vi "Bar Page.vi"() -> ()   [LabVIEW 2017, in "3D Bar.lvclass"]
uses:
  <vilib>/Math Plots/3D Math Plots/3D Bar/3D Bar/3D Bar.lvclass
  <vilib>/Math Plots/3D Math Plots/3D Bar/3D Bar/Typedef/3D Bar Property Array.ctl
  <vilib>/Math Plots/3D Math Plots/3D Bar/3D Bar/Typedef/3D Bar Property.ctl
  <vilib>/Math Plots/3D Math Plots/3D Plot/3D Plot/Typedef/Line Type.ctl
  <vilib>/Math Plots/3D Math Plots/3D Plot/3D Plot/Typedef/Dialog State.ctl
  <vilib>/Math Plots/3D Math Plots/3D Plot/3D Plot/Typedef/Temp Scene State.ctl
  <vilib>/Math Plots/3D Math Plots/3D Plot/3D Plot/Typedef/Temp Scene Property Action.ctl
  <vilib>/Math Plots/3D Math Plots/3D Plot/3D Plot/3D Plot.lvclass
panel:
  in  "Bar Mode":u16(ring) caption="Bar mode" items=["Detach", "Group", "Stack"]
  in  "Line Style":u16(ring) caption="Line style"
  in  "Antialiasing":bool
  in  "Line Width":sgl=0.001 caption="Line width" min=0.001 step=1
  in  "Line Color":u32(colorbox) caption="Line color"
  in  "Color and Name":cluster{"Label Color":u32, "String":string}[](array[cluster]) caption="Color and name"
  in  "Bar Size":sgl=1.0 caption="Bar size" min=0.001 max=1 step=0.1
  out "Bar Property Out":T1
  in  "Bar Property In":T1
  in  "YZ Plane Projection":bool caption="YZ plane projection"
  in  "XZ Plane Projection":bool caption="XZ plane projection"
  in  "XY Plane Projection":bool caption="XY plane projection"
  in  "Coordinate System":u16(ring) caption="Coordinate system" items=["Cartesian", "Cylindrical", "Spherical"]
  in  "Plot Opacity":sgl(slide) caption="Plot opacity(%)" min=0 max=100 scale=0.0..100.0
  in  "Plot List":i32(listbox)
  in  "Move Down":bool
  in  "Move Up":bool
  in  "Delete":bool
  in  "New":bool
  in  "Event Registration":refnum<event-registration>
  # "Bar"
  # "General"
  # "Projection"
  # "Bar"
  # "Outline"
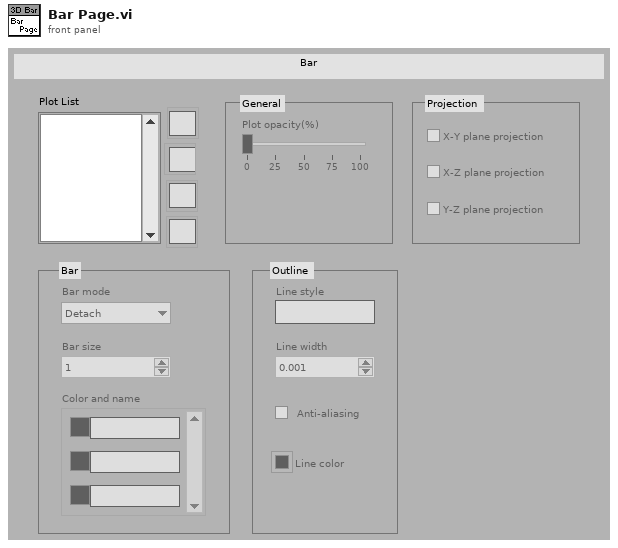
[diagram p1: front panel]
types:
  T1 = typedef "3D Bar.lvclass/3D Bar Property Array.ctl" = T2[]
  T2 = typedef "3D Bar.lvclass/3D Bar Property.ctl" = cluster{"General Property":cluster{"Plot Name":string, "Coordinate System":enum16{"Cartesian", "Cylindrical", "Spherical"}, "Opacity":sgl}, "Projection Property":cluster{"Draw XY":bool, "Draw YZ":bool, "Draw XZ":bool}, "Plot Property":cluster{"Line Style":T3, "Line Width":sgl, "Line Color":u32, "Antialiasing":bool}, "Bar Property":cluster{"Bar Mode":enum16{"Detach", "Group", "Stack"}, "Bar Width":sgl, "Color Pair Array":cluster{"Color":u32, "String":string}[]}}
  T3 = typedef "3D Plot.lvclass/Line Type.ctl" = enum16{"None", "Solid", "Dash", "Dot", "Dash Dot"}
  T4 = typedef "3D Plot.lvclass/Dialog State.ctl" = enum16{"Initialize", "Read Porperty", "Write Property", "Idle", "Exit"}
  T5 = typedef "3D Plot.lvclass/Temp Scene State.ctl" = enum16{"Create", "Update Scene", "Get Plot Representation", "Destory"}
  T6 = typedef "3D Plot.lvclass/Temp Scene Property Action.ctl" = enum16{"Graph Property", "Light Property", "Axis Property", "Value Pair Property", "Format Property", "Cursor Property", "Plot Specific Property"}
  T7 = typedef "3D Plot.lvclass/Multiplot Representation.ctl" = cluster{"Plot Represention Array":T8[], "Max Range":T9}
  T8 = typedef "3D Plot.lvclass/Plot Representation.ctl" = cluster{"Plot ID":i32, "Plot Range":T9, "Mesh Data":T10, "Dimension":cluster{"X Dimension":i32, "Y Dimension":i32}, "Ramp Range":T9}
  T9 = typedef "3D Plot.lvclass/Range Clusters.ctl" = cluster{"X Range":cluster{"Max X":sgl, "Min X":sgl}, "Y Range":cluster{"Max Y":sgl, "Min Y":sgl}, "Z Range":cluster{"Max Z":sgl, "Min Z":sgl}}
  T10 = typedef "3D Plot.lvclass/Mesh Data.ctl" = cluster{"Index Array":u32[], "Vertex Array":cluster{"X":sgl, "Y":sgl, "Z":sgl}[], "Normal Array":cluster{"X":sgl, "Y":sgl, "Z":sgl}[], "Color Index Array":i32[]}
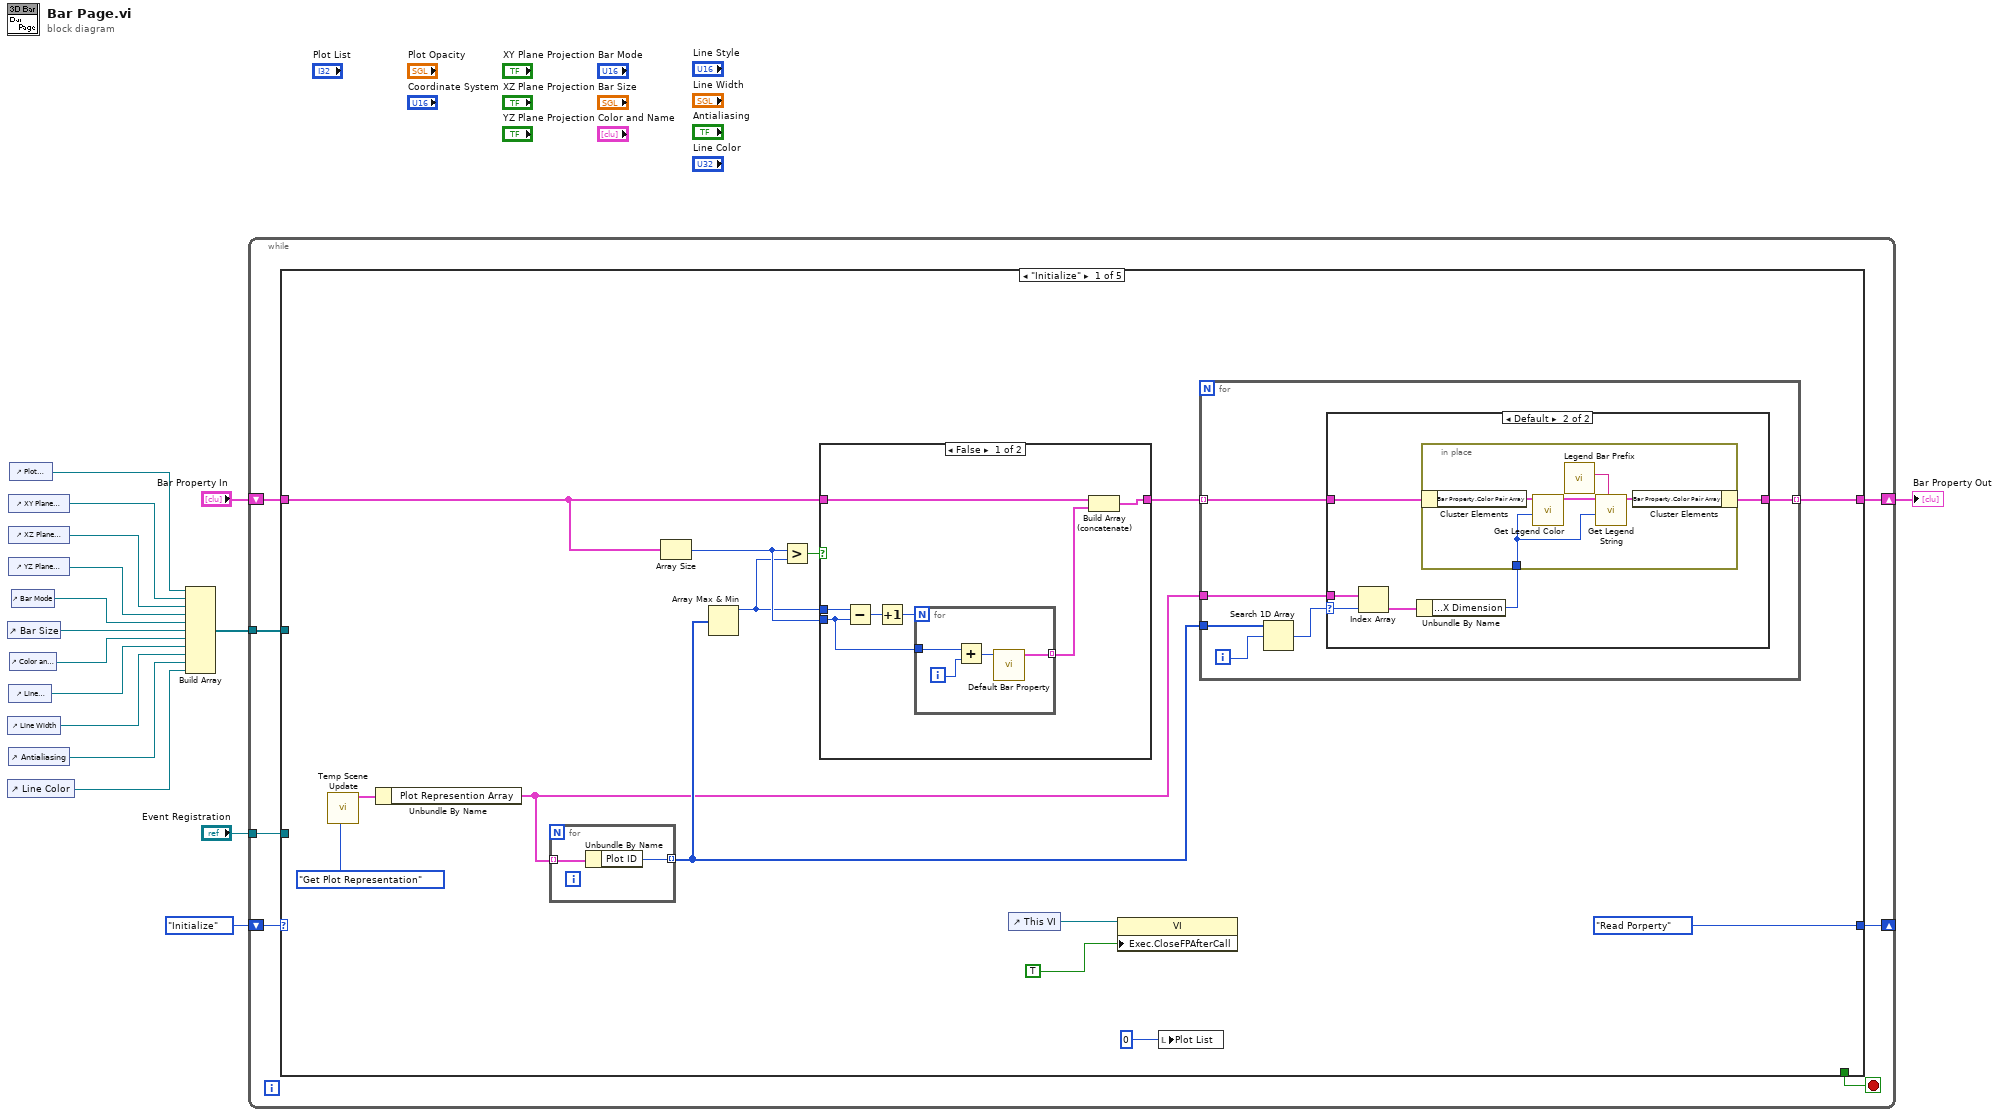
[diagram p0: block diagram]
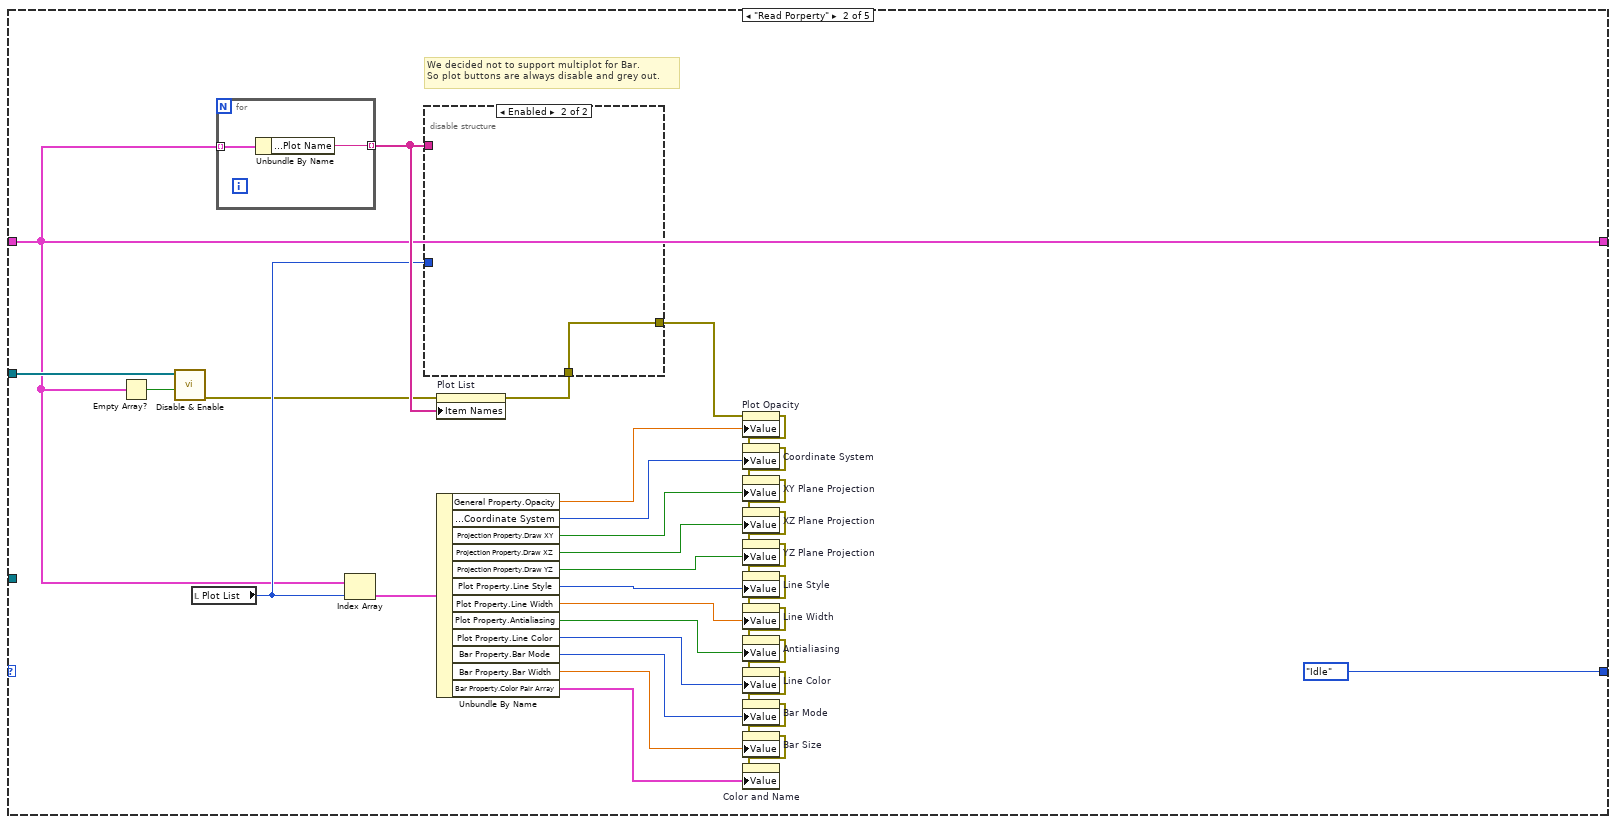
[diagram p4: hidden frame]
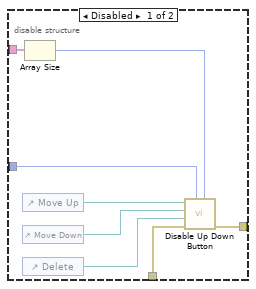
[diagram p5: hidden frame]
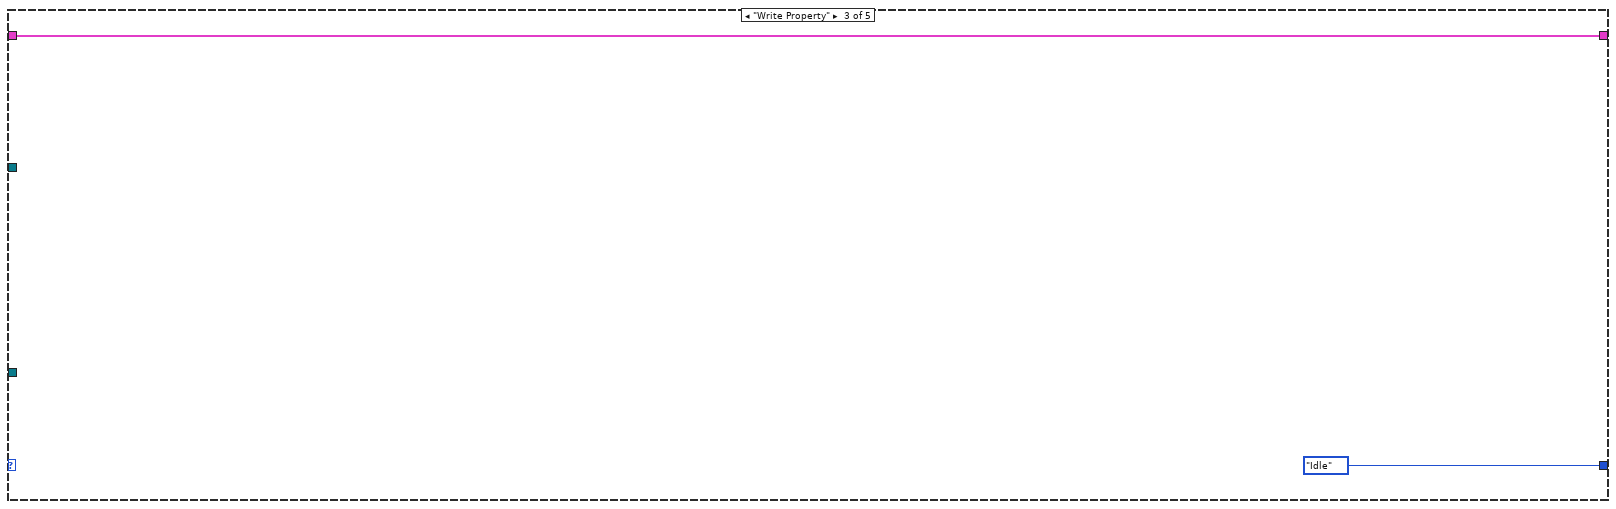
[diagram p6: hidden frame]
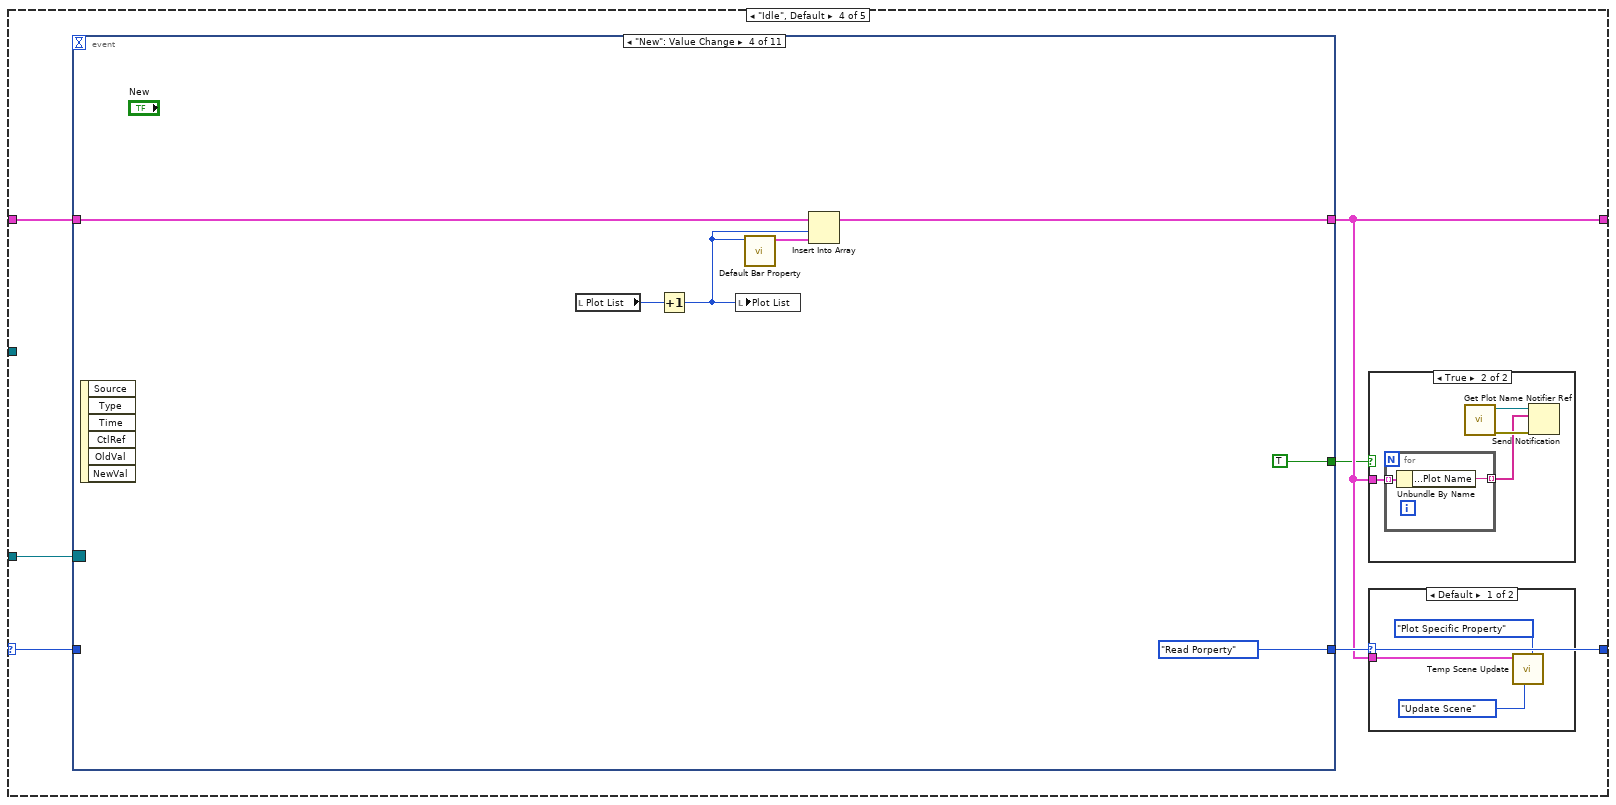
[diagram p7: hidden frame]
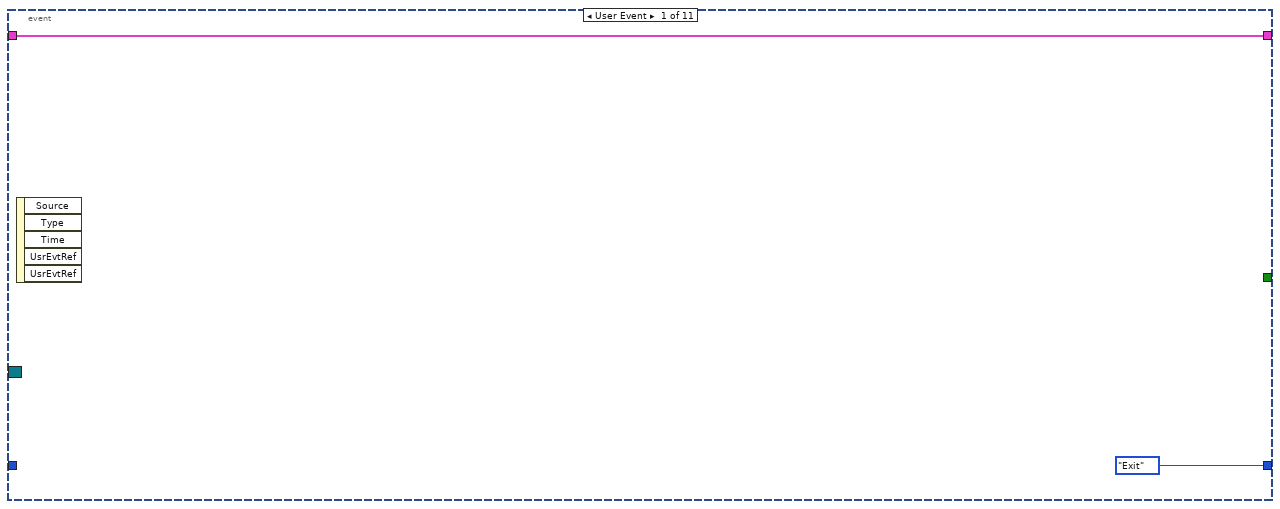
[diagram p10: hidden frame]
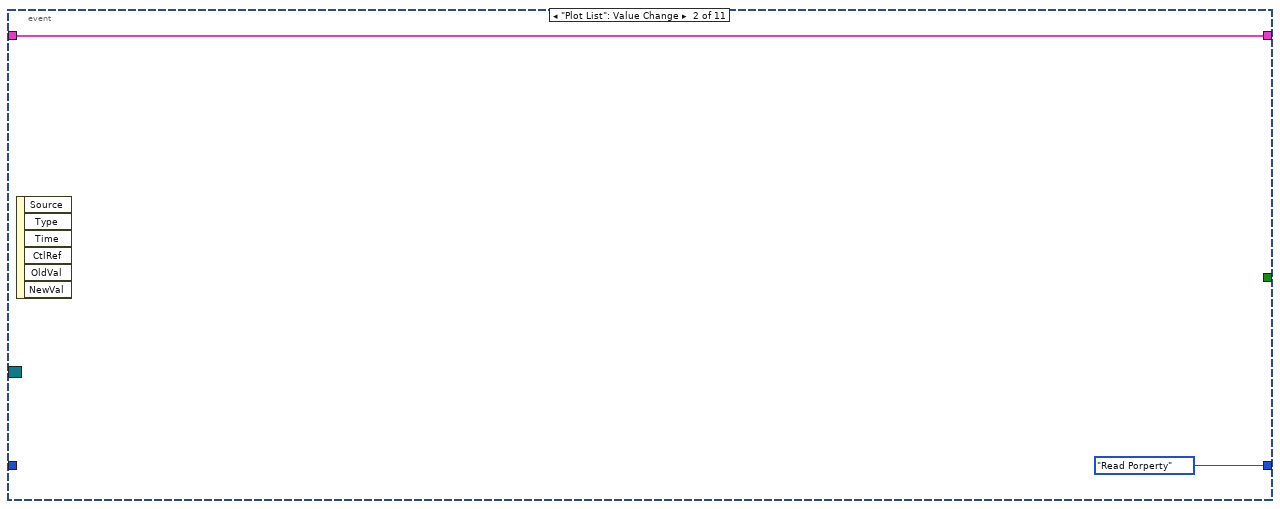
[diagram p11: hidden frame]
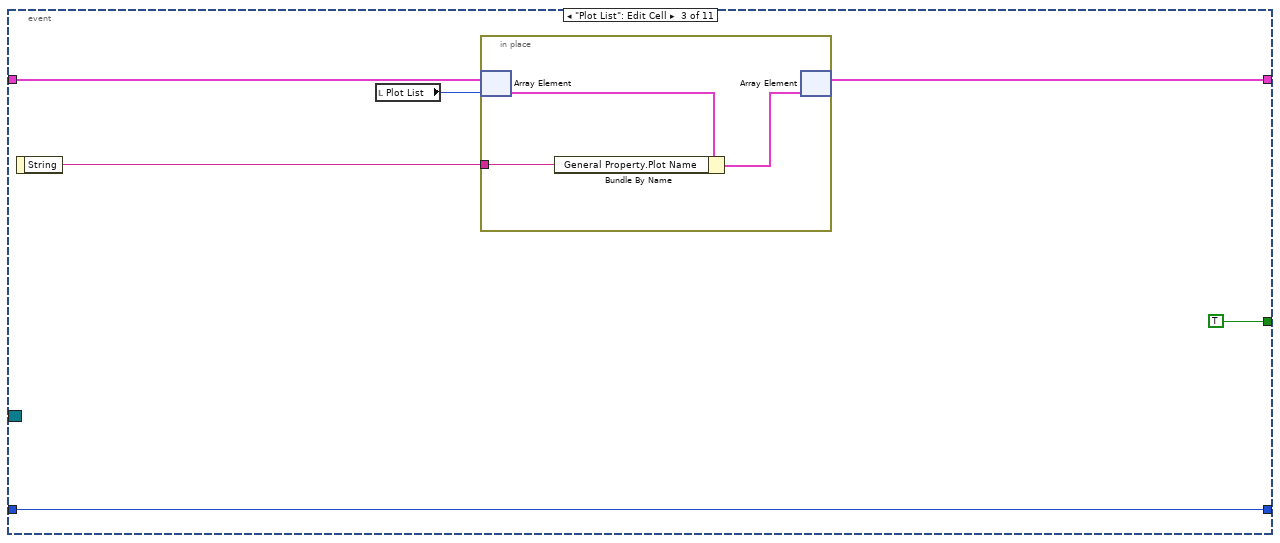
[diagram p12: hidden frame]
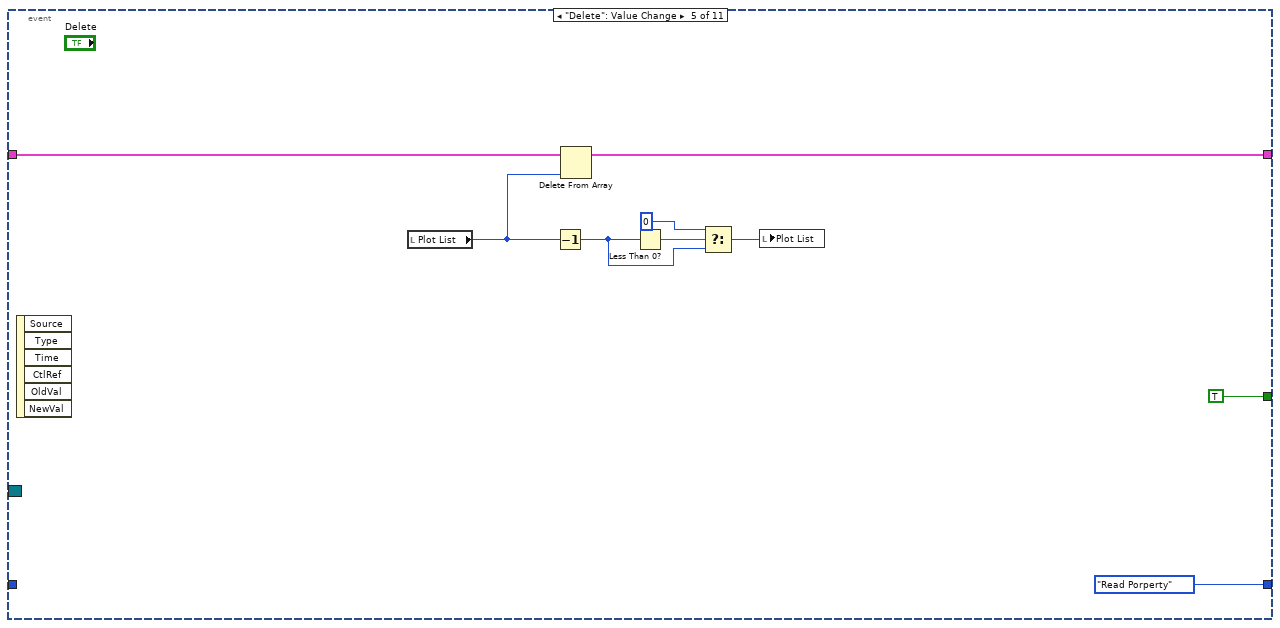
[diagram p13: hidden frame]
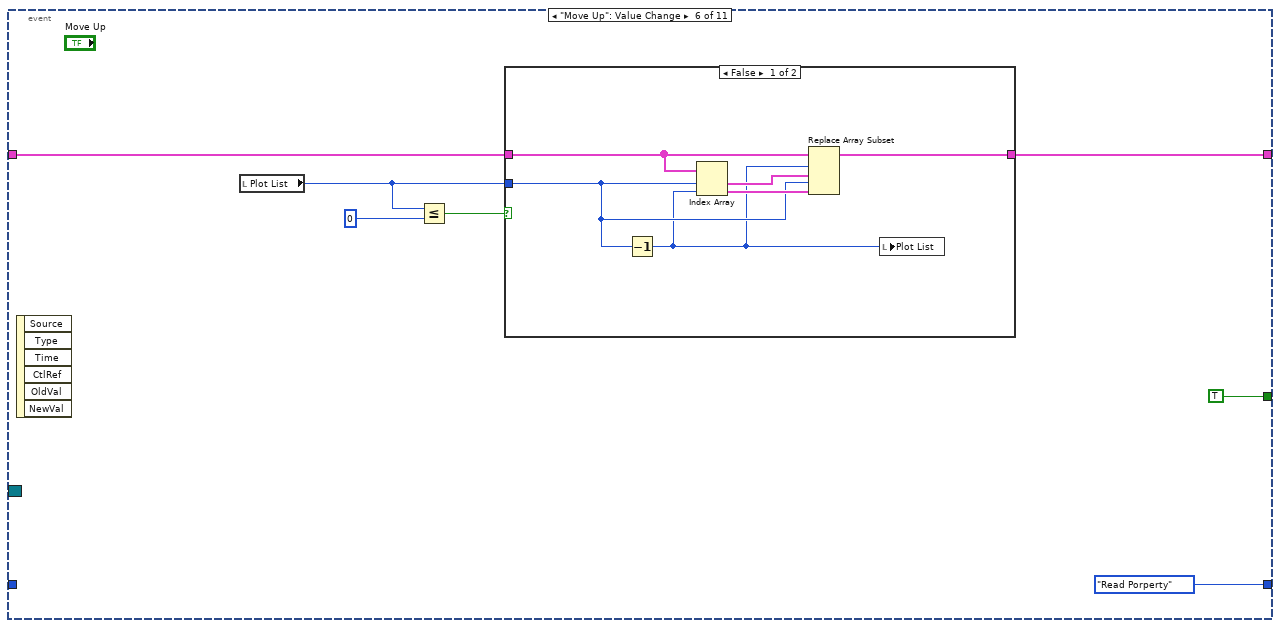
[diagram p14: hidden frame]
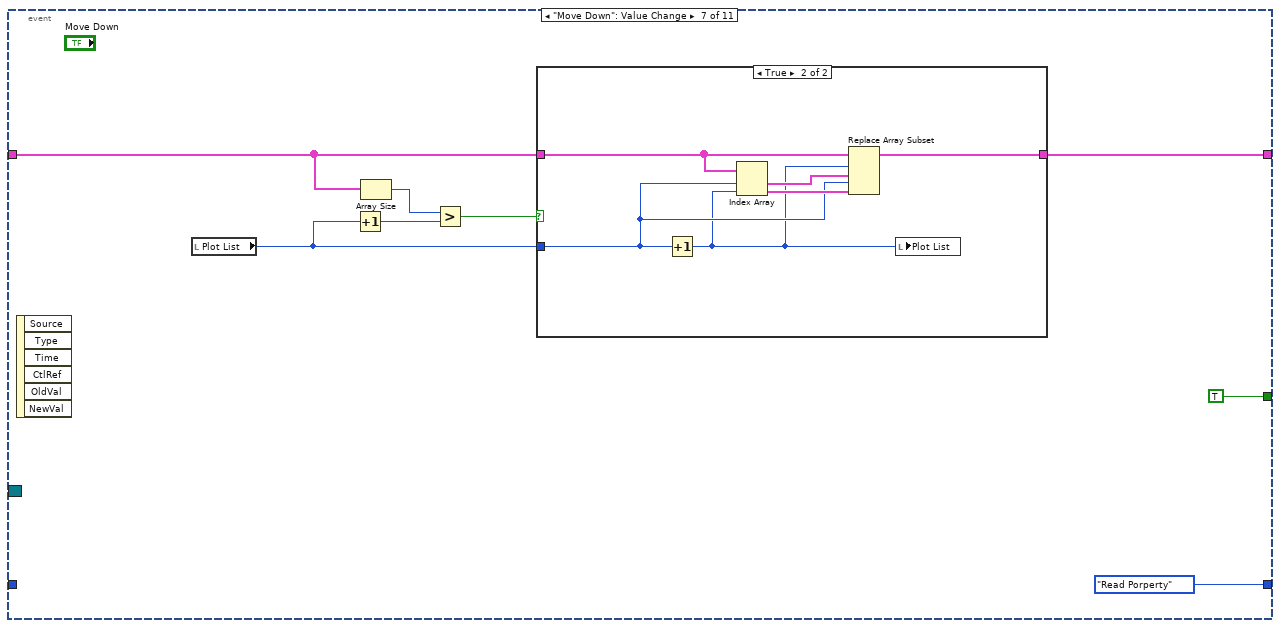
[diagram p16: hidden frame]
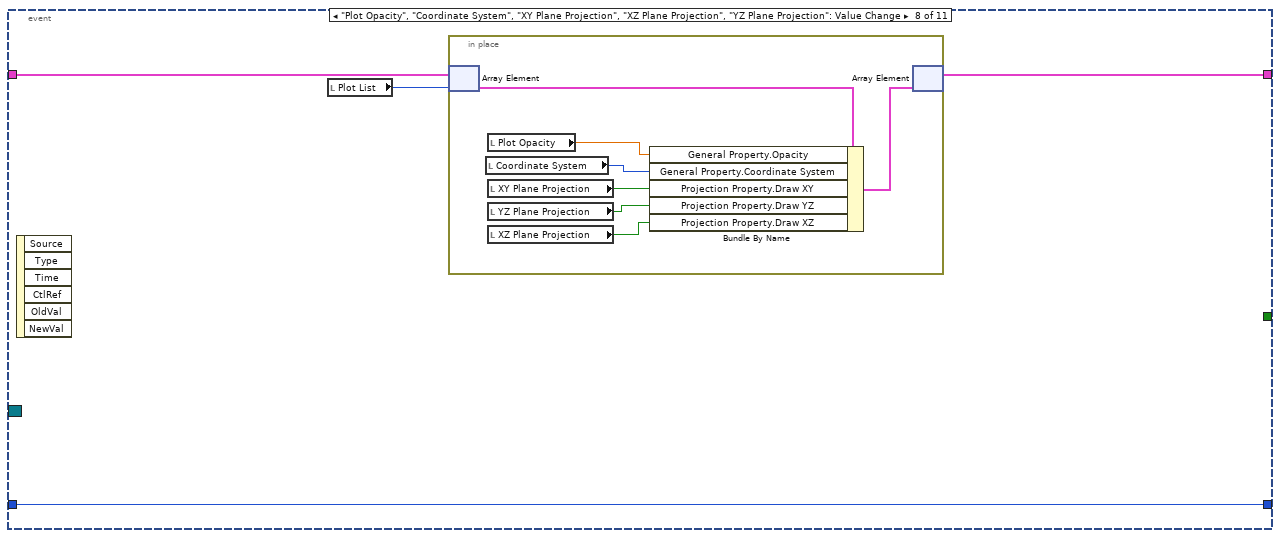
[diagram p18: hidden frame]
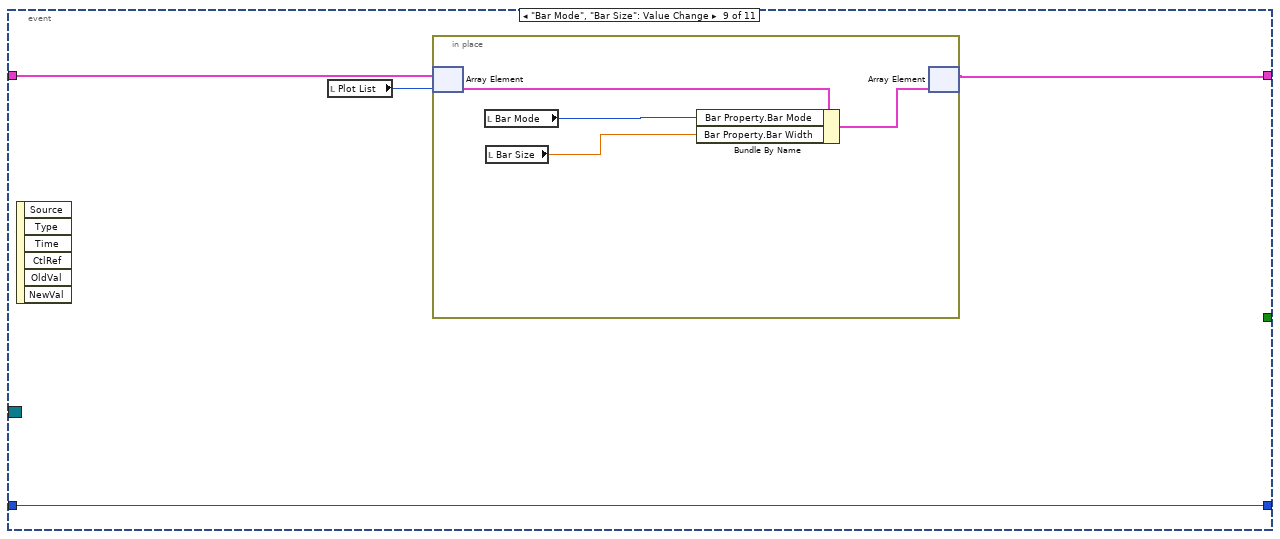
[diagram p19: hidden frame]
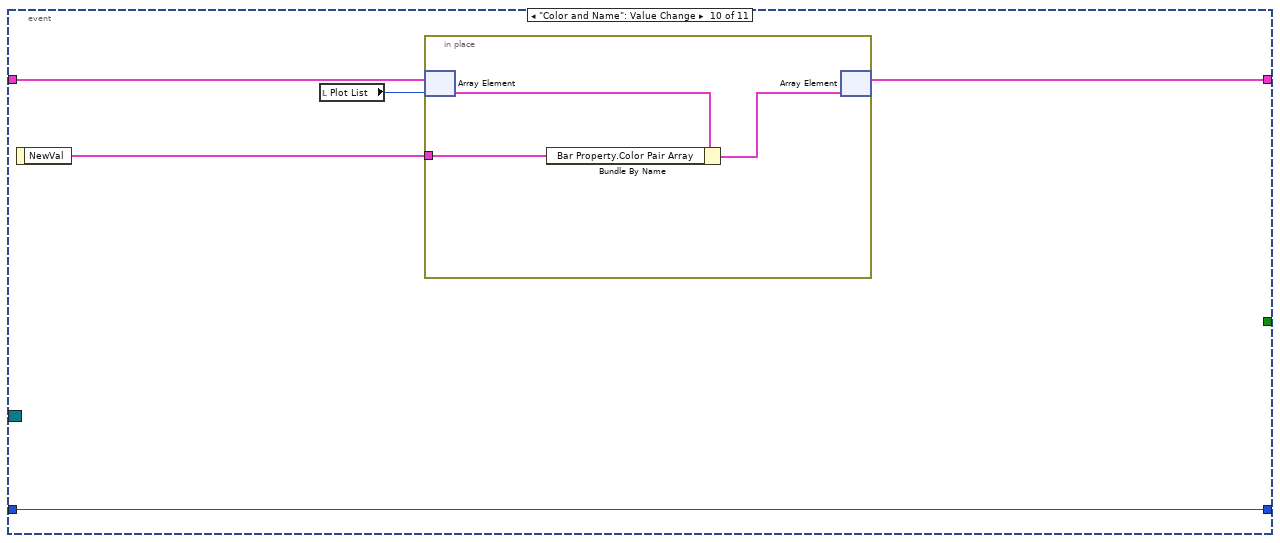
[diagram p20: hidden frame]
diagram:
  n1 = control-ref of="Bar Size"() -> (w7:refnum<vi>)
  n2 = control-ref of="Line Width"() -> (w4:refnum<vi>)
  n3 = control-ref of="Line Color"() -> (w2:refnum<vi>)
  n4 = control-ref of="XY Plane Projection"() -> (w11:refnum<vi>)
  n5 = control-ref of="XZ Plane Projection"() -> (w10:refnum<vi>)
  n6 = control-ref of="YZ Plane Projection"() -> (w9:refnum<vi>)
  n7 = control-ref of="Line Style"() -> (w5:refnum<vi>)
  n8 = control-ref of="Antialiasing"() -> (w3:refnum<vi>)
  n9 = control-ref of="Plot Opacity"() -> (w12:refnum<vi>)
  n10 = control-ref of="Color and Name"() -> (w6:refnum<vi>)
  n11 = control-ref of="Bar Mode"() -> (w8:refnum<vi>)
  n12 = Build Array(w12, w11, w10, w9, w8, w7, w6, w5, w4, w3, w2) -> (w1:refnum<vi>[])
  n13 = while {
    shift-right: [w22] -> w13
    shift-left: "Bar Property In" -> [w23]
    shift-right: [w18] -> _
    shift-left: Dialog_State."Initialize" -> [w21]
    tunnel: "Event Registration" -> [w19]
    tunnel: w1 -> [w17]
    stop <- w20 stop-if-true
    n14 = case shown="\"Initialize\"" w21 {
      selector: w21 -> [_ _ _ w119 _]
      tunnel: w23 -> [w28 w95 w114 w121 w226]
      tunnel: [w33 w95 w114 w117 w226] -> w22
      tunnel: [Dialog_State."Read Porperty" Dialog_State."Idle" Dialog_State."Idle" w118 Dialog_State."Exit"] -> w18
      tunnel: [_ _ _ _ TRUE] -> w20
      tunnel: w19 -> [_ _ _ w120 _]
      tunnel: w17 -> [_ w96 _ _ _]
      frame "Initialize" {
        n15 = call <vilib>:"Temp Scene Update.vi"("State"=Temp_Scene_State."Get Plot Representation") -> ("Multiplot Representation"=w26:T7)  [unwired: 5 in, 5 out]
        n16 = Unbundle By Name(w26) -> ("Plot Represention Array"=w24:T8[])
        n17 = for {
          tunnel: w24 -> [w51] mode=indexing
          tunnel: [w50] -> w25 mode=indexing
          n18 = Unbundle By Name(w51) -> ("Plot ID"=w50:i32)
        }
        n19 = Array Size(array=w28) -> (size(s)=w30:i32)
        n20 = Array Max & Min(array=w25) -> (max value=w29:i32)  [unwired: 3 out]
        n21 = Greater?(x=w30, y=w29) -> (0:w31:bool)
        n22 = case shown="False" w31 {
          tunnel: [w42 w49] -> w27
          tunnel: w28 -> [w44 w49]
          tunnel: w30 -> [w38 _]
          tunnel: w29 -> [w39 _]
          frame False {
            n23 = Subtract(x=w39, y=w38) -> (x-y=w41:i32)
            n24 = Increment(x=w41) -> (x+1=w40:i32)
            n25 = for {
              N: w40 -> [_]
              tunnel: w38 -> [w47]
              tunnel: [w45] -> w43 mode=indexing
              i -> [w48]
              n26 = Add(x=w47, y=w48) -> (x+y=w46:i32)
              n27 = call <vilib>:"Default Bar Property.vi"("Plot ID"=w46) -> ("Default Property"=w45:T2)  [unwired: 10 out]
            }
            n28 = Build Array (concatenate)(w44, w43) -> (w42:T1)
          }
          frame True {
          }
        }
        n29 = control-ref of="This VI"() -> (w36:refnum<vi>)
        n30 = property class="VI"(reference=w36, "Exec.CloseFPAfterCall"=TRUE ("Execution:Close After Call")) -> ()  [unwired: 1 in, 2 out]
        n31 = local write "Plot List"(0 ("Plot List")) -> ()
        n32 = for {
          tunnel: w27 -> [w57] mode=indexing
          tunnel: w24 -> [w55]
          tunnel: [w56] -> w33 mode=indexing
          tunnel: w25 -> [w54]
          i -> [w53]
          n33 = Search 1D Array(1D array=w54, element=w53) -> (index of element=w52:i32)  [unwired: 1 out]
          n34 = case shown="Default" w52 {
            selector: w52 -> [_ w59]
            tunnel: w57 -> [w58 w63]
            tunnel: [w58 w62] -> w56
            tunnel: w55 -> [_ w61]
            frame -1 {
            }
            frame Default {
              n35 = Index Array(array=w61, index=w59) -> (element=w60:T8)
              n36 = Unbundle By Name(w60) -> ("Dimension.X Dimension"=w64:i32)
              n37 = in-place {
                in-place-border: w64 -> [w66]
                n38 = in-place-cluster #1(w63) -> ("Bar Property.Color Pair Array"=w68:cluster{"Color":u32, "String":string}[])
                n39 = call <vilib>:"Get Legend Color.vi"("Pair Array Length"=w66, "Color Pair Array In"=w68) -> ("Color Pair Array Out"=w69:cluster{"Color":u32, "String":string}[])  [unwired: 9 out]
                n40 = call <vilib>:"Legend Bar Prefix.vi"() -> ("Prefix Out"=w65:string)  [unwired: 11 out]
                n41 = call <vilib>:"Get Legend String.vi"("Initial String"=w65, "Pair Array Length"=w66, "Color Pair Array In"=w69) -> ("Color Pair Array Out"=w67:cluster{"Color":u32, "String":string}[])  [unwired: 8 out]
                n42 = in-place-cluster #1("Bar Property.Color Pair Array"=w67) -> (w62:T2)
              }
            }
          }
        }
      }
      frame "Read Porperty" {
        # "We decided not to support multiplot for Bar.\nSo plot buttons are always disable and grey out."
        n43 = Empty Array?(array=w95) -> (empty?=w97:bool)
        n44 = call <vilib>:"Disable & Enable.vi"("Disabled?"=w97, "Control Ref Array"=w96) -> ("error out"=w94:errorcluster)  [unwired: 1 in, 8 out]
        n45 = local read "Plot List"() -> (w98:i32)
        n46 = for {
          tunnel: w95 -> [w113] mode=indexing
          tunnel: [w112] -> w100 mode=indexing
          n47 = Unbundle By Name(w113) -> ("General Property.Plot Name"=w112:string)
        }
        n48 = Index Array(array=w95, index=w98) -> (element=w101:T2)
        n49 = property on="Plot List" class="LstBox (strict)"(error in=w94, "Item Names"=w100) -> (error out=w99:errorcluster)  [unwired: 1 in, 1 out]
        n50 = disable-structure shown="Enabled" {
          disable-tunnel: w100 -> [w106 _]
          disable-tunnel: w99 -> [w105 w111]
          disable-tunnel: w98 -> [w104 _]
          disable-tunnel: [w103 w111] -> w70
          frame Disabled {
            n51 = control-ref of="Move Up"() -> (w108:refnum<vi>)
            n52 = control-ref of="Move Down"() -> (w109:refnum<vi>)
            n53 = control-ref of="Delete"() -> (w110:refnum<vi>)
            n54 = Array Size(array=w106) -> (size(s)=w107:i32)
            n55 = call <vilib>:"Disable Up Down Button.vi"("Length"=w107, "Index"=w104, "error in (no error)"=w105, "Delete Ref"=w110, "Move Down Ref"=w109, "Move Up Ref"=w108) -> ("error out"=w103:errorcluster)  [unwired: 5 out]
          }
          frame Enabled {
          }
        }
        n56 = Unbundle By Name(w101) -> ("General Property.Opacity"=w82:sgl, "General Property.Coordinate System"=w81:enum16{"Cartesian", "Cylindrical", "Spherical"}, "Projection Property.Draw XY"=w80:bool, "Projection Property.Draw XZ"=w79:bool, "Projection Property.Draw YZ"=w78:bool, "Plot Property.Line Style"=w77:T3, "Plot Property.Line Width"=w76:sgl, "Plot Property.Antialiasing"=w75:bool, "Plot Property.Line Color"=w74:u32, "Bar Property.Bar Mode"=w73:enum16{"Detach", "Group", "Stack"}, "Bar Property.Bar Width"=w72:sgl, "Bar Property.Color Pair Array"=w71:cluster{"Color":u32, "String":string}[])
        n57 = property on="Plot Opacity" class="Slide (strict)"(error in=w70, "Value"=w82) -> (error out=w93:errorcluster)  [unwired: 1 in, 1 out]
        n58 = property on="Coordinate System" class="Ring (strict)"(error in=w93, "Value"=w81) -> (error out=w92:errorcluster)  [unwired: 1 in, 1 out]
        n59 = property on="XY Plane Projection" class="Bool (strict)"(error in=w92, "Value"=w80) -> (error out=w91:errorcluster)  [unwired: 1 in, 1 out]
        n60 = property on="XZ Plane Projection" class="Bool (strict)"(error in=w91, "Value"=w79) -> (error out=w90:errorcluster)  [unwired: 1 in, 1 out]
        n61 = property on="YZ Plane Projection" class="Bool (strict)"(error in=w90, "Value"=w78) -> (error out=w89:errorcluster)  [unwired: 1 in, 1 out]
        n62 = property on="Line Style" class="Ring (strict)"(error in=w89, "Value"=w77) -> (error out=w88:errorcluster)  [unwired: 1 in, 1 out]
        n63 = property on="Line Width" class="DigNum (strict)"(error in=w88, "Value"=w76) -> (error out=w87:errorcluster)  [unwired: 1 in, 1 out]
        n64 = property on="Antialiasing" class="Bool (strict)"(error in=w87, "Value"=w75) -> (error out=w86:errorcluster)  [unwired: 1 in, 1 out]
        n65 = property on="Line Color" class="ColBox"(error in=w86, "Value"=w74) -> (error out=w85:errorcluster)  [unwired: 1 in, 1 out]
        n66 = property on="Bar Mode" class="Ring (strict)"(error in=w85, "Value"=w73) -> (error out=w84:errorcluster)  [unwired: 1 in, 1 out]
        n67 = property on="Bar Size" class="DigNum (strict)"(error in=w84, "Value"=w72) -> (error out=w83:errorcluster)  [unwired: 1 in, 1 out]
        n68 = property on="Color and Name" class="Arr (strict)"(error in=w83, "Value"=w71) -> ()  [unwired: 1 in, 2 out]
      }
      frame "Write Property" {
      }
      frame "Idle", Default {
        n69 = event shown="[3] \"New\": Value Change" {
          selector: w120 -> [_ _ _ _ _ _ _ _ _ _ _]
          dyn-events: _ -> [_ _ _ _ _ _ _ _ _ _ _]
          timeout: _ -> [_ _ _ _ _ _ _ _ _ _ _]
          tunnel: w121 -> [w132 w134 w138 w148 w157 w162 w176 w190 w201 w212 w217]
          tunnel: [w132 w134 w137 w147 w158 w161 w175 w189 w200 w211 w216] -> w117
          tunnel: [Dialog_State."Exit" Dialog_State."Read Porperty" w136 Dialog_State."Read Porperty" Dialog_State."Read Porperty" Dialog_State."Read Porperty" Dialog_State."Read Porperty" w192 w203 w208 w219] -> w118
          tunnel: w119 -> [_ _ w136 _ _ _ _ w192 w203 w208 w219]
          tunnel: [_ _ TRUE TRUE TRUE TRUE TRUE _ _ _ _] -> w116
          event User Event {
            n70 = event-data() -> ()  [unwired: 6 out]
          }
          event "Plot List": Value Change {
            n71 = event-data() -> ()  [unwired: 7 out]
          }
          event "Plot List": Edit Cell {
            n72 = event-data() -> ("String"=w139:string)  [unwired: 1 out]
            n73 = local read "Plot List"() -> (w140:i32)
            n74 = in-place {
              in-place-border: w139 -> [w141]
              n75 = in-place-array #2(w138, w140) -> (w143:T2)
              n76 = Bundle By Name(cluster=w143, "General Property.Plot Name"=w141) -> (w142:T2)
              n77 = in-place-array #2(w142) -> (w137:T1)  [unwired: 1 out]
            }
          }
          event "New": Value Change {
            n78 = event-data() -> ()  [unwired: 7 out]
            n79 = local read "Plot List"() -> (w149:i32)
            n80 = Increment(x=w149) -> (x+1=w145:i32)
            n81 = local write "Plot List"(w145) -> ()
            n82 = call <vilib>:"Default Bar Property.vi"("Plot ID"=w145) -> ("Default Property"=w144:T2)  [unwired: 10 out]
            n83 = Insert Into Array(array=w148, index=w145, new element=w144) -> (w147:T1)
          }
          event "Delete": Value Change {
            n84 = event-data() -> ()  [unwired: 7 out]
            n85 = local read "Plot List"() -> (w153:i32)
            n86 = Decrement(x=w153) -> (x-1=w154:i32)
            n87 = Delete From Array(array=w157, index=w153) -> (array with subset deleted=w158:T1)  [unwired: 1 in, 1 out]
            n88 = Less Than 0?(x=w154) -> (x < 0?=w156:bool)
            n89 = Select(t=0, s=w156, f=w154) -> (s? t:f=w152:i32)
            n90 = local write "Plot List"(w152) -> ()
          }
          event "Move Up": Value Change {
            n91 = event-data() -> ()  [unwired: 7 out]
            n92 = local read "Plot List"() -> (w163:i32)
            n93 = Less Or Equal?(x=w163, y=0) -> (x <= y?=w165:bool)
            n94 = case shown="False" w165 {
              tunnel: w162 -> [w170 w173]
              tunnel: [w169 w173] -> w161
              tunnel: w163 -> [w168 _]
              frame False {
                n95 = Decrement(x=w168) -> (x-1=w167:i32)
                n96 = Index Array(array=w170, index #1=w168, index #2=w167) -> (element #1=w172:T2, element #2=w171:T2)
                n97 = Replace Array Subset(array=w170, new element #1=w172, index #1=w167, new element #2=w171, index #2=w168) -> (w169:T1)
                n98 = local write "Plot List"(w167) -> ()
              }
              frame True {
                # "List value is less or equal to 0.\nThe active item is in the top of the list."
              }
            }
          }
          event "Move Down": Value Change {
            n99 = event-data() -> ()  [unwired: 7 out]
            n100 = local read "Plot List"() -> (w177:i32)
            n101 = Increment(x=w177) -> (x+1=w179:i32)
            n102 = Array Size(array=w176) -> (size(s)=w178:i32)
            n103 = Greater?(x=w178, y=w179) -> (0:w180:bool)
            n104 = case shown="True" w180 {
              tunnel: w176 -> [w182 w186]
              tunnel: [w182 w185] -> w175
              tunnel: w177 -> [_ w184]
              frame False {
                # "List value +1 is not less array length.\nThe active item is in the buttom of the list."
              }
              frame True {
                n105 = Increment(x=w184) -> (x+1=w183:i32)
                n106 = Index Array(array=w186, index #1=w184, index #2=w183) -> (element #1=w188:T2, element #2=w187:T2)
                n107 = Replace Array Subset(array=w186, new element #1=w188, index #1=w183, new element #2=w187, index #2=w184) -> (w185:T1)
                n108 = local write "Plot List"(w183) -> ()
              }
            }
          }
          event "Plot Opacity", "Coordinate System", "XY Plane Projection", "XZ Plane Projection", "YZ Plane Projection": Value Change {
            n109 = event-data() -> ()  [unwired: 7 out]
            n110 = local read "Plot List"() -> (w191:i32)
            n111 = in-place {
              n112 = in-place-array #3(w190, w191) -> (w195:T2)
              n113 = local read "Coordinate System"() -> (w193:u16)
              n114 = local read "Plot Opacity"() -> (w199:sgl)
              n115 = local read "XY Plane Projection"() -> (w198:bool)
              n116 = local read "YZ Plane Projection"() -> (w196:bool)
              n117 = local read "XZ Plane Projection"() -> (w197:bool)
              n118 = Bundle By Name(cluster=w195, "General Property.Opacity"=w199, "General Property.Coordinate System"=w193, "Projection Property.Draw XY"=w198, "Projection Property.Draw YZ"=w196, "Projection Property.Draw XZ"=w197) -> (w194:T2)
              n119 = in-place-array #3(w194) -> (w189:T1)  [unwired: 1 out]
            }
          }
          event "Bar Mode", "Bar Size": Value Change {
            n120 = event-data() -> ()  [unwired: 7 out]
            n121 = local read "Plot List"() -> (w202:i32)
            n122 = in-place {
              n123 = in-place-array #4(w201, w202) -> (w205:T2)
              n124 = local read "Bar Mode"() -> (w207:u16)
              n125 = local read "Bar Size"() -> (w206:sgl)
              n126 = Bundle By Name(cluster=w205, "Bar Property.Bar Mode"=w207, "Bar Property.Bar Width"=w206) -> (w204:T2)
              n127 = in-place-array #4(w204) -> (w200:T1)  [unwired: 1 out]
            }
          }
          event "Color and Name": Value Change {
            n128 = event-data() -> ("NewVal"=w210:cluster{"Label Color":u32, "String":string}[])  [unwired: 1 out]
            n129 = local read "Plot List"() -> (w209:i32)
            n130 = in-place {
              in-place-border: w210 -> [w213]
              n131 = in-place-array #5(w212, w209) -> (w215:T2)
              n132 = Bundle By Name(cluster=w215, "Bar Property.Color Pair Array"=w213) -> (w214:T2)
              n133 = in-place-array #5(w214) -> (w211:T1)  [unwired: 1 out]
            }
          }
          event "Line Style", "Line Width", "Antialiasing", "Line Color": Value Change {
            n134 = event-data() -> ()  [unwired: 7 out]
            n135 = local read "Plot List"() -> (w218:i32)
            n136 = in-place {
              n137 = in-place-array #6(w217, w218) -> (w222:T2)
              n138 = local read "Line Style"() -> (w225:u16)
              n139 = local read "Antialiasing"() -> (w223:bool)
              n140 = local read "Line Color"() -> (w220:u32)
              n141 = local read "Line Width"() -> (w224:sgl)
              n142 = Bundle By Name(cluster=w222, "Plot Property.Line Style"=w225, "Plot Property.Line Width"=w224, "Plot Property.Antialiasing"=w223, "Plot Property.Line Color"=w220) -> (w221:T2)
              n143 = in-place-array #6(w221) -> (w216:T1)  [unwired: 1 out]
            }
          }
        }
        n144 = case shown="True" w116 {
          tunnel: w117 -> [_ w122]
          frame False {
          }
          frame True {
            n145 = for {
              tunnel: w122 -> [w127] mode=indexing
              tunnel: [w126] -> w123 mode=indexing
              n146 = Unbundle By Name(w127) -> ("General Property.Plot Name"=w126:string)
            }
            n147 = call <vilib>:"Get Plot Name Notifier Ref.vi"() -> ("error out"=w125:errorcluster, "Plot Names Notifier Ref"=w124:refnum<notifier>)  [unwired: 1 in, 9 out]
            n148 = Send Notification(notification=w123, notifier=w124, error in (no error)=w125) -> ()  [unwired: 2 out]
          }
        }
        n149 = case shown="Default" w118 {
          tunnel: w117 -> [w130 _]
          frame Default {
            n150 = call <vilib>:"Temp Scene Update.vi"("Property Name"=Temp_Scene_Property_Action."Plot Specific Property", "State"=Temp_Scene_State."Update Scene", "Property In"=w130) -> ()  [unwired: 3 in, 6 out]
          }
          frame "Exit" {
          }
        }
      }
      frame "Exit" {
      }
    }
  }
  "Bar Property Out" <- w13
